vi "miniScanSelector.vi"(0 "X-Y-Z coordinates":T1 {"Z stop" format="%#_6f"; "Z start" format="%#_6f"; "ROI group ID" format="%#_6f"; "Laser Power (%)" format="%#_6f"; "Zoom" format="%#_6f"; "Frame Size" format="%#_6f"; "Number of lines" format="%#_6f"; "Composite ID" format="%#_6f"; "Angle (deg)" format="%#_6f"; "ROI Time (ns)" format="%#_6f"; "ROI ID" format="%#_6f"; "Pixels in ROI" format="%#_6f"; "ROI index" format="%#_6f"; "Y stop" format="%#_6f"; "X stop" format="%#_6f"; "X start" format="%#_6f"; "Y start" format="%#_6f"}, 3 "index":i32, 5 "Main zoom":dbl, 9 "FrameSize":i32) -> (14 "Norm X Start":dbl, 15 "Norm Y Start":dbl, 16 "Norm Z Start":dbl, 17 "Norm X Stop":dbl, 18 "Norm Y Stop":dbl, 19 "Norm Z Stop":dbl)   [LabVIEW 2017]
uses:
  User Interface/Visualisation/Functional Imaging Viewer/Typedefs/ROI parameters data type.ctl
panel:
  in  "Temporary offset (0)":dbl format="%#_13g"
  # "<--- For vertical miniscans only"
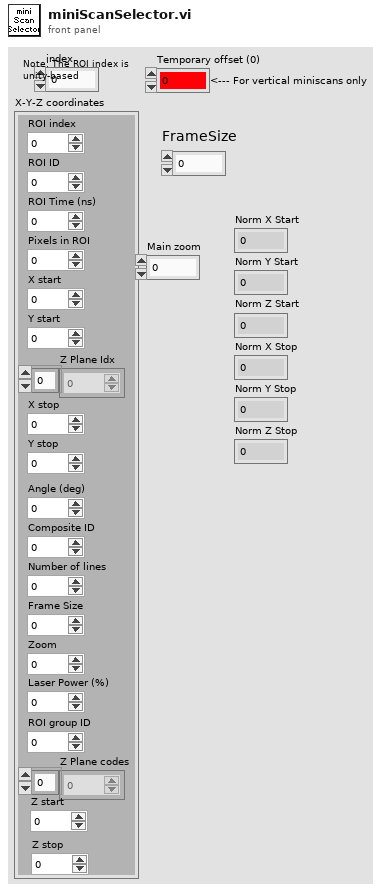
[diagram p1: front panel]
types:
  T1 = typedef "ROI parameters data type.ctl" = cluster{"ROI index":dbl, "ROI ID":dbl, "ROI Time (ns)":dbl, "Pixels in ROI":dbl, "X start":dbl, "Y start":dbl, "X stop":dbl, "Y stop":dbl, "Angle (deg)":dbl, "Composite ID":dbl, "Number of lines":dbl, "Frame Size":dbl, "Zoom":dbl, "Laser Power (%)":dbl, "ROI group ID":dbl, "Z Plane Idx":i32[], "Z Plane codes":u8[], "Z start":dbl, "Z stop":dbl}
  T2 = typedef "Angle type.ctl" = enum16{"Horisontal (0 deg)", "Vertical (90 deg)", "Any other angle"}
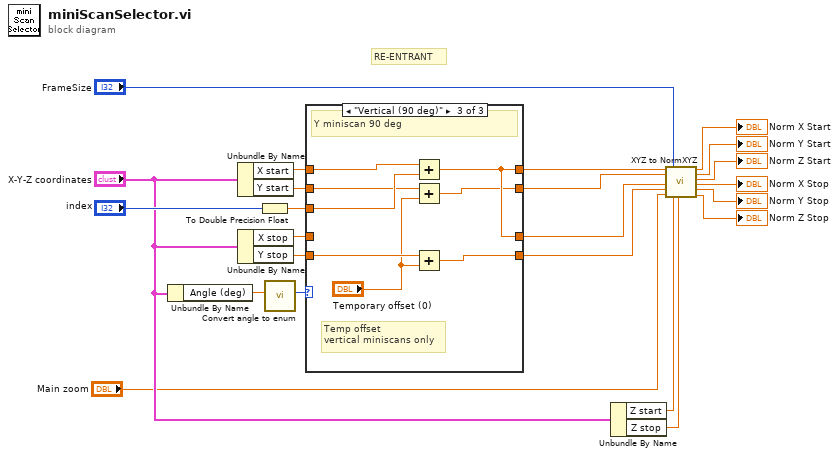
[diagram p0: block diagram]
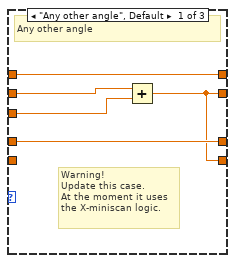
[diagram p2: hidden frame]
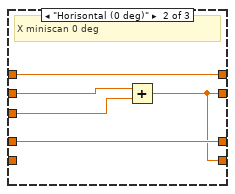
[diagram p3: hidden frame]
diagram:
  # "RE-ENTRANT"
  n1 = Unbundle By Name("X-Y-Z coordinates") -> ("Angle (deg)"=w3:dbl)
  n2 = Unbundle By Name("X-Y-Z coordinates") -> ("X start"=w22:dbl, "Y start"=w21:dbl)
  n3 = Unbundle By Name("X-Y-Z coordinates") -> ("X stop"=w20:dbl, "Y stop"=w19:dbl)
  n4 = To Double Precision Float(number="index") -> (double precision float=w18:dbl)
  n5 = call "Convert angle to enum.vi"("Angle"=w3) -> ("Miniscan angle"=w2:T2)  [unwired: 10 in]
  n6 = case shown="\"Vertical (90 deg)\"" w2 {
    tunnel: [w28 w33 w40] -> w17
    tunnel: w22 -> [w28 w33 w39]
    tunnel: w21 -> [w25 w30 w38]
    tunnel: [w24 w29 w37] -> w16
    tunnel: w20 -> [w27 w32 _]
    tunnel: [w27 w32 w40] -> w15
    tunnel: w19 -> [_ _ w36]
    tunnel: [w24 w29 w35] -> w14
    tunnel: w18 -> [w26 w31 w41]
    frame "Any other angle", Default {
      # "Warning!\nUpdate this case.\nAt the moment it uses\nthe X-miniscan logic."
      # "Any other angle"
      n7 = Add(x=w25, y=w26) -> (x+y=w24:dbl)
    }
    frame "Horisontal (0 deg)" {
      # "X miniscan 0 deg"
      n8 = Add(x=w30, y=w31) -> (x+y=w29:dbl)
    }
    frame "Vertical (90 deg)" {
      # "Temp offset\nvertical miniscans only"
      # "Y miniscan 90 deg"
      n9 = Add(x=w39, y=w41) -> (x+y=w40:dbl)
      n10 = Add(x=w38, y="Temporary offset (0)") -> (x+y=w37:dbl)
      n11 = Add(x=w36, y="Temporary offset (0)") -> (x+y=w35:dbl)
    }
  }
  n12 = Unbundle By Name("X-Y-Z coordinates") -> ("Z start"=w13:dbl, "Z stop"=w12:dbl)
  n13 = call "XYZ to NormXYZ.vi"("X start"=w17, "Y start"=w16, "X stop"=w15, "Y stop"=w14, "Zoom (either ref or main zoom)"="Main zoom", "FrameSize"="FrameSize", "Z start"=w13, "Z stop"=w12) -> ("Norm X Start"=→"Norm X Start":dbl, "Norm Y Start"=→"Norm Y Start":dbl, "Norm Z Start"=→"Norm Z Start":dbl, "Norm X Stop"=→"Norm X Stop":dbl, "Norm Y Stop"=→"Norm Y Stop":dbl, "Norm Z Stop"=→"Norm Z Stop":dbl)  [unwired: 6 in]
